vi "Digital Write 1 Channel.vi"(8 "error constant":errorcluster, 9 "Value":bool=TRUE, 10 "Channel":i32, 11 "NI-DAQ.lvclass":refnum<class "NI-DAQ.lvclass">) -> (0 "error IO":errorcluster, 3 "NI-DAQ.lvclass 2":refnum<class "NI-DAQ.lvclass">)   [LabVIEW 2021, in "NI-DAQ.lvclass"]
uses:
  NI-DAQ.lvclass
  NI-DAQ.lvclass/NI-DAQ.ctl
  <vilib>/Utility/file.llb/Read Delimited Spreadsheet (string).vi
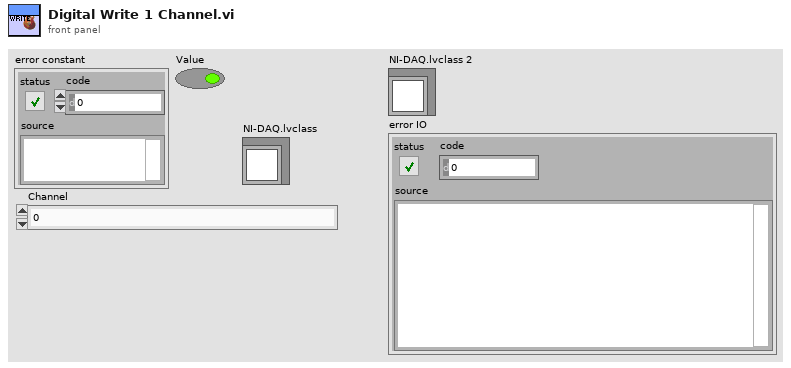
[diagram p1: front panel]
types:
  T1 = typedef "File Paths.ctl" = cluster{"Glue Pattern Folder":path, "Carrier Tray Folder":path, "Pick Up Tool Fixture Folder":path, "Components Folder":path, "Bellows Tool Offset.txt":path, "Pick Up Tool Offset.txt":path, "Dispense Tip Offset.txt":path, "Log Files":path, "Gantry Assembly Map.txt":path, "Syringe and offset map.txt":path, "Controllers Folder":path, "Local dbase config":path}
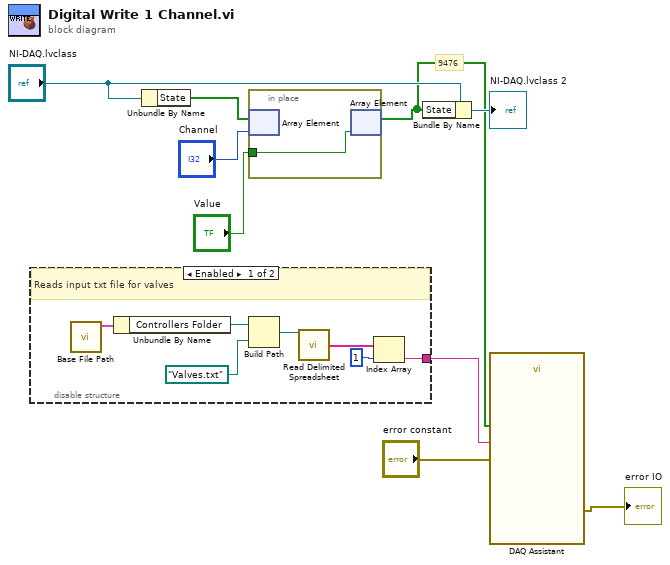
[diagram p0: block diagram]
diagram:
  # "9476"
  n1 = disable-structure shown="Enabled" {
    disable-tunnel: [w10 _] -> w1
    frame Enabled {
      # "Reads input txt file for valves"
      n2 = call "Base File Path.vi"() -> ("Paths Out"=w16:T1)  [unwired: 11 in]
      n3 = Unbundle By Name(w16) -> ("Controllers Folder"=w15:path)
      n4 = Build Path(base path=w15, name or relative path=path "Valves.txt") -> (appended path=w13:path)
      n5 = call-poly <vilib>:"Read Delimited Spreadsheet.vi"("file path (dialog if empty)"=w13) -> ("first row"=w12:string[])  [unwired: 9 in, 5 out]
      n6 = Index Array(array=w12, index=1 ("dimension size")) -> (element=w10:string)
    }
    frame Disabled {
    }
  }
  n7 = Unbundle By Name("NI-DAQ.lvclass") -> ("State"=w5:bool[])
  n8 = in-place {
    in-place-border: "Value" -> [w17]
    n9 = in-place-array #1(w5, "Channel") -> ()  [unwired: 1 out]
    n10 = in-place-array #1(w17) -> (w4:bool[])  [unwired: 1 out]
  }
  n11 = Bundle By Name(cluster="NI-DAQ.lvclass", "State"=w4) -> (→"NI-DAQ.lvclass 2":refnum<class "NI-DAQ.lvclass">)
  n12 = call "DAQ Assistant"("data"=w4, "error in"="error constant", "device name"=w1) -> ("error out"=→"error IO":errorcluster)  [unwired: 15 in, 1 out]
